vi "dfd_FXP Casting (scaler).vi"(5 "quantization settings":T4={"source"=6, "wl"=1, "iwl"=1, "overflow mode"=enum."Saturation", "rounding mode"=enum."Nearest", "signed?"=TRUE} {"source" items=["Coef a/k"=0, "Coef b/v"=7, "Input"=1, "Output"=2, "Multiplicand"=3, "Product"=4, "Sum"=5, "Delay"=6, "Gain"=8]}, 6 "filtering statistics in":T3(array[cluster]) {"statistics information"."min value" format="%.2f"; "statistics information"."max value" format="%.2f"; "Quantizer Source" items=["Coefficients a/k"=0, "Coefficients b/v"=7, "Input"=1, "Output"=2, "Multiplicand"=3, "Product"=4, "Sum"=5, "Delay"=6]}, 9 "value in":dbl format="%.2f") -> (0 "filtering statistics out":T3(array[cluster]) {"statistics information"."min value" format="%.2f"; "statistics information"."max value" format="%.2f"; "Quantizer Source" items=["Coefficients a/k"=0, "Coefficients b/v"=7, "Input"=1, "Output"=2, "Multiplicand"=3, "Product"=4, "Sum"=5, "Delay"=6]}, 2 "statistics information":T2 {"min value" format="%.2f"; "max value" format="%.2f"}, 3 "value out":dbl format="%.2f")   [LabVIEW 2017, in "NI_DigFilter_FXP.lvlib"]
uses:
  <vilib>/addons/Digital Filter Design/NI_DigFilter_FXP.lvlib
  <vilib>/addons/Digital Filter Design/_Objects.llb/dfd_Internal Quantization Settings.ctl
  <vilib>/addons/Digital Filter Design/_Objects.llb/dfd_Internal Quantization Srcs.ctl
  <vilib>/addons/Digital Filter Design/_Objects.llb/DFD FXP Statistics Data.ctl
  <vilib>/addons/Digital Filter Design/_Objects.llb/DFD Quantization Sources.ctl
  <vilib>/addons/Digital Filter Design/FXPLib.llb/dfd_FXP Overflow (scaler).vi
  <vilib>/addons/Digital Filter Design/FXPLib.llb/dfd_FXP Quantization (scaler).vi
  <vilib>/addons/Digital Filter Design/NI_DigFilterLicensed.lvlib
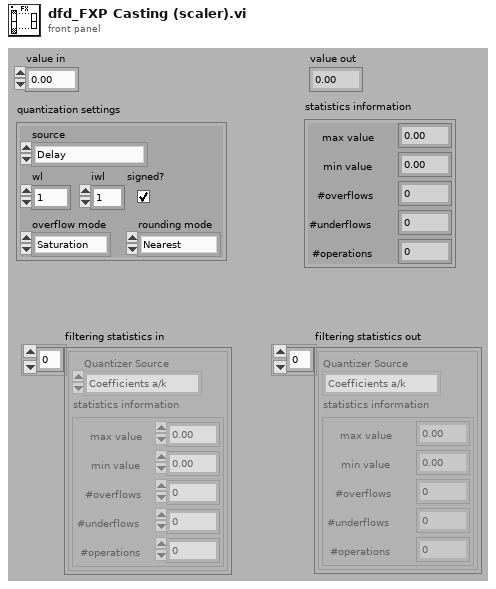
[diagram p1: front panel]
types:
  T1 = typedef "NI_DigFilterLicensed.lvlib/DFD Quantization Sources.ctl" = u16
  T2 = typedef "NI_DigFilterLicensed.lvlib/DFD FXP Statistics Data.ctl" = cluster{"max value":ext, "min value":ext, "#overflows":i32, "#underflows":i32, "#operations":i32}
  T3 = cluster{"Quantizer Source":T1, "statistics information":T2}[]
  T4 = typedef "NI_DigFilterLicensed.lvlib/dfd_Internal Quantization Settings.ctl" = cluster{"source":T5, "wl":i16, "iwl":i16, "overflow mode":enum16{"Saturation", "Wrap"}, "rounding mode":enum16{"Nearest", "Truncation"}, "signed?":bool}
  T5 = typedef "NI_DigFilterLicensed.lvlib/dfd_Internal Quantization Srcs.ctl" = u16
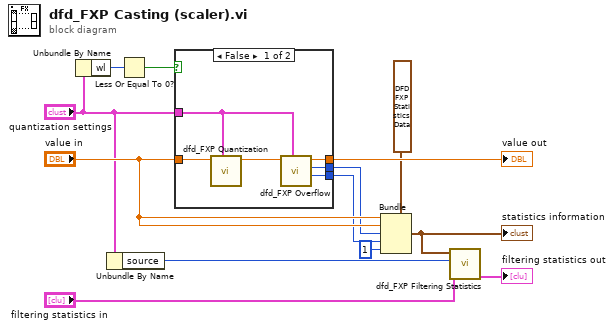
[diagram p0: block diagram]
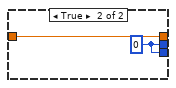
[diagram p2: hidden frame]
diagram:
  n1 = Unbundle By Name("quantization settings") -> ("wl"=w10:i16)
  n2 = Unbundle By Name("quantization settings") -> ("source"=w3:T5)
  n3 = Less Or Equal To 0?(x=w10) -> (x <= 0?=w5:bool)
  n4 = case shown="False" w5 {
    tunnel: [w19 w21] -> w13
    tunnel: "value in" -> [w18 w21]
    tunnel: "quantization settings" -> [w17 _]
    tunnel: [w15 w20] -> w8
    tunnel: [w14 w20] -> w7
    frame False {
      n5 = call-poly <vilib>:"dfd_FXP Quantization.vi"("quantization settings"=w17, "value in"=w18) -> ("value out"=w16:dbl)  [unwired: 6 out]
      n6 = call-poly <vilib>:"dfd_FXP Overflow.vi"("quantization settings"=w17, "value in"=w16) -> ("# underflow"=w14:i32, "# overflow"=w15:i32, "value out"=w19:dbl)  [unwired: 4 out]
    }
    frame True {
      w20 = 0 ("#overflow")
    }
  }
  "value out" <- w13
  n7 = Bundle(cluster=T2 {"max value"=0.0, "min value"=0.0, "#overflows"=0, "#underflows"=0, "#operations"=0} ("statistics information"), "max value"="value in", "min value"="value in", "#overflows"=w8, "#underflows"=w7, "#operations"=1) -> (w11:T2)
  "statistics information" <- w11
  n8 = call <vilib>:"dfd_FXP Filtering Statistics.vi"("filtering statistics in"="filtering statistics in", "source"=w3, "new data"=w11) -> ("filtering statistics out"=→"filtering statistics out":T3)  [unwired: 1 in, 7 out]
